vi "프로젝트 test용.vi"   [LabVIEW 2021]
uses:
  <vilib>/addons/database/Connection.llb/DB Tools Open Connec (String).vi
  <vilib>/addons/database/NI_Database_API.lvlib
types:
  T1 = typedef "NI_Database_API.lvlib/Conn ObjectReference.ctl" = refnum<k1>
  T2 = cluster{"[0]":string, "[1]":string, "[2]":string}
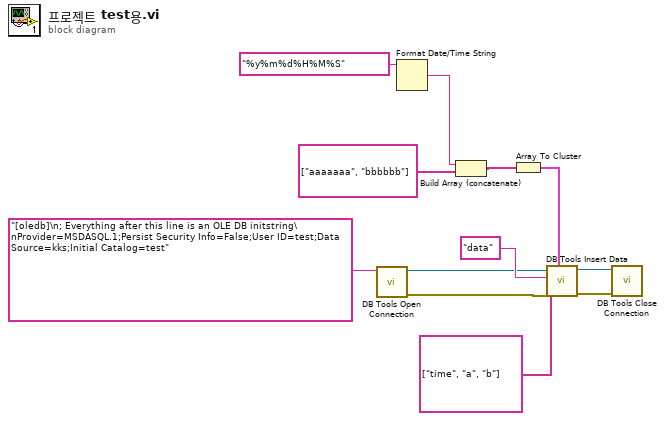
[diagram p0: block diagram]
diagram:
  n1 = call-poly <vilib>:"DB Tools Open Connection.vi"("connection information"="[oledb]\n; Everything after this line is an OLE DB initstring\nProvider=MSDASQL.1;Persist Security Info=False;User ID=test;Data Source=kks;Initial Catalog=test") -> ("error out"=w1:errorcluster, "connection reference"=w2:T1)  [unwired: 7 in]
  n2 = Format Date/Time String(time format string (%c)="%y%m%d%H%M%S" ("시간 포맷 문자열 (%c)")) -> (date/time string=w10:string)  [unwired: 2 in]
  n3 = Build Array (concatenate)(w10, string[] ["aaaaaaa", "bbbbbb"] ("배열")) -> (w9:string[])
  n4 = Array To Cluster(array=w9) -> (cluster=w12:T2)
  n5 = call <vilib>:"DB Tools Insert Data.vi"("data"=w12, "error in (no error)"=w1, "columns"=string[] ["time", "a", "b"], "table"="data", "connection reference"=w2) -> ("error out"=w3:errorcluster, "connection reference out"=w4:T1)  [unwired: 5 in]
  n6 = call <vilib>:"DB Tools Close Connection.vi"("error in (no error)"=w3, "connection reference"=w4) -> ()  [unwired: 5 in, 1 out]
